vi "Untitled 5 (SubVI).vi"(10 "Boolean":bool, 11 "Boolean 2":bool) -> (3 "Numeric":i32)   [LabVIEW 2017]
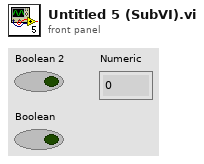
[diagram p1: front panel]
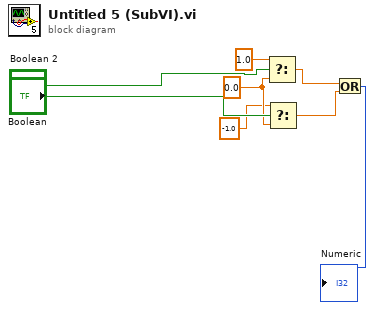
[diagram p0: block diagram]
diagram:
  w2 = 0.0 ("t")
  n1 = Select(t=1.0, s="Boolean 2", f=w2) -> (s? t:f=w4:dbl)
  n2 = Select(t=-1.0, s="Boolean", f=w2) -> (s? t:f=w3:dbl)
  n3 = Or(x=w4, y=w3) -> (x .or. y?=→"Numeric":i32)
